vi "3090仪器参数上传.vi"(11 "错误输入（无错误）":errorcluster) -> (15 "error out":errorcluster)   [LabVIEW 2016, in "数据传输系统.lvlib"]
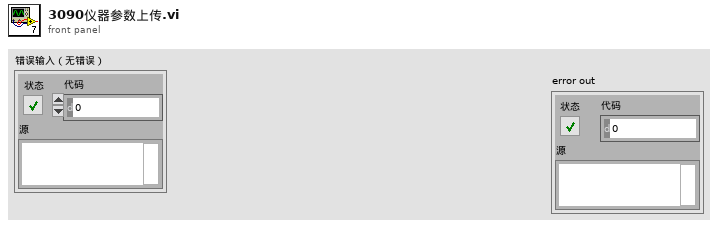
[diagram p1: front panel]
types:
  T1 = cluster{"氨氮仪器参数索引起始时间":string, "总磷仪器参数索引起始时间":string, "总氮仪器参数索引起始时间":string, "CODMn仪器参数索引起始时间":string, "CODCr仪器参数索引起始时间":string, "DO仪器参数索引起始时间":string, "PH仪器参数索引起始时间":string, "比电导率仪器参数索引起始时间":string, "水温仪器参数索引起始时间":string, "浊度仪器参数索引起始时间":string, "叶绿素a仪器参数索引起始时间":string, "藻密度仪器参数索引起始时间":string, "ORP仪器参数索引起始时间":string}
  T2 = cluster{"[0]":string, "[1]":string, "[2]":string, "[3]":string, "[4]":string, "[5]":string, "[6]":string, "[7]":string, "[8]":string, "[9]":string, "[10]":string, "[11]":string, "[12]":string}
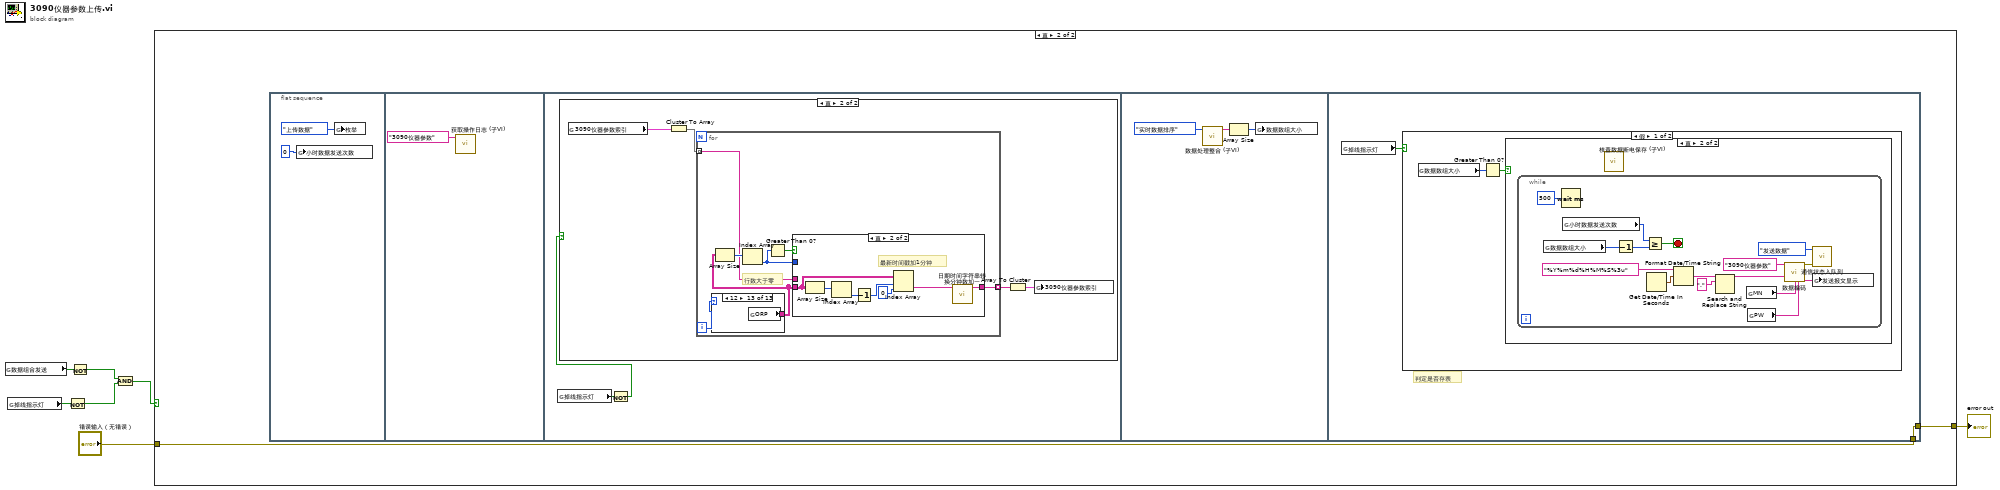
[diagram p0: block diagram]
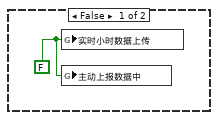
[diagram p2: hidden frame]
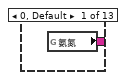
[diagram p4: hidden frame]
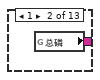
[diagram p5: hidden frame]
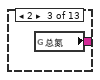
[diagram p6: hidden frame]
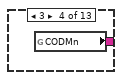
[diagram p7: hidden frame]
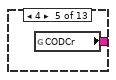
[diagram p8: hidden frame]
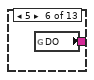
[diagram p9: hidden frame]
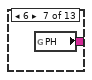
[diagram p10: hidden frame]
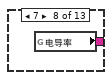
[diagram p11: hidden frame]
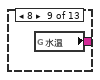
[diagram p12: hidden frame]
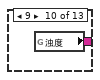
[diagram p13: hidden frame]
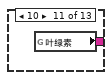
[diagram p14: hidden frame]
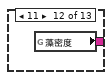
[diagram p15: hidden frame]
diagram:
  n1 = global read "断电保存全局.vi" "数据组合发送"() -> (w4:bool)
  n2 = global read "全局 数据发送重叠.vi" "掉线指示灯"() -> (w7:bool)
  n3 = Not(x=w7) -> (.not. x?=w2:bool)
  n4 = Not(x=w4) -> (.not. x?=w3:bool)
  n5 = And(x=w3, y=w2) -> (x .and. y?=w1:bool)
  n6 = case shown="真" w1 {
    tunnel: [_ w10] -> w6
    tunnel: "错误输入（无错误）" -> [_ w9]
    frame False {
      w8 = FALSE ("小时数据上传")
      n7 = global write "全局1.vi" "实时小时数据上传"(w8) -> ()
      n8 = global write "全局 数据发送重叠.vi" "主动上报数据中"(w8) -> ()
    }
    frame True {
      n9 = flat-sequence {
        tunnel: [w51] -> w10
        tunnel: w9 -> [w51]
        frame #0 {
          n10 = global write "全局 小时数据发送次数.vi" "小时数据发送次数"(0 ("小时数据发送次数")) -> ()
          n11 = global write "全局1.vi" "枚举"(enum16{"返回请求应答", "上传数据", "返回执行结果"}."上传数据" ("枚举")) -> ()
        }
        frame #1 {
          n12 = call "获取操作日志 (子VI).vi"("table输入"="3090仪器参数") -> ()  [unwired: 11 in]
        }
        frame #2 {
          n13 = global read "全局 数据发送重叠.vi" "掉线指示灯"() -> (w15:bool)
          n14 = Not(x=w15) -> (.not. x?=w14:bool)
          n15 = case shown="真" w14 {
            frame False {
            }
            frame True {
              n16 = global read "全局 时间2.vi" "3090仪器参数索引"() -> (w19:T1)
              n17 = Cluster To Array(cluster=w19) -> (array=w18:string[])
              n18 = for {
                tunnel: [w23] -> w16 mode=indexing
                tunnel: w18 -> [w22] mode=indexing
                i -> [w21]
                # "行数大于零"
                n19 = case shown="12" w21 {
                  tunnel: [w27 w28 w29 w30 w31 w32 w33 w34 w35 w36 w37 w38 w39] -> w20
                  frame 0, Default {
                    n20 = global read "全局 所有参数.vi" "氨氮"() -> (w27:string[][])
                  }
                  frame 1 {
                    n21 = global read "全局 所有参数.vi" "总磷"() -> (w28:string[][])
                  }
                  frame 2 {
                    n22 = global read "全局 所有参数.vi" "总氮"() -> (w29:string[][])
                  }
                  frame 3 {
                    n23 = global read "全局 所有参数.vi" "CODMn"() -> (w30:string[][])
                  }
                  frame 4 {
                    n24 = global read "全局 所有参数.vi" "CODCr"() -> (w31:string[][])
                  }
                  frame 5 {
                    n25 = global read "全局 所有参数.vi" "DO"() -> (w32:string[][])
                  }
                  frame 6 {
                    n26 = global read "全局 所有参数.vi" "PH"() -> (w33:string[][])
                  }
                  frame 7 {
                    n27 = global read "全局 所有参数.vi" "电导率"() -> (w34:string[][])
                  }
                  frame 8 {
                    n28 = global read "全局 所有参数.vi" "水温"() -> (w35:string[][])
                  }
                  frame 9 {
                    n29 = global read "全局 所有参数.vi" "浊度"() -> (w36:string[][])
                  }
                  frame 10 {
                    n30 = global read "全局 所有参数.vi" "叶绿素"() -> (w37:string[][])
                  }
                  frame 11 {
                    n31 = global read "全局 所有参数.vi" "藻密度"() -> (w38:string[][])
                  }
                  frame 12 {
                    n32 = global read "全局 所有参数.vi" "ORP"() -> (w39:string[][])
                  }
                }
                n33 = Array Size(array=w20) -> (size(s)=w25:i32[])
                n34 = Index Array(array=w25) -> (element=w24:i32)  [unwired: 1 in]
                n35 = Greater Than 0?(x=w24) -> (x > 0?=w26:bool)
                n36 = case shown="真" w26 {
                  tunnel: w24 -> [_ _]
                  tunnel: w20 -> [_ w44]
                  tunnel: [w40 w41] -> w23
                  tunnel: w22 -> [w40 _]
                  frame False {
                  }
                  frame True {
                    # "最新时间戳加1分钟"
                    n37 = Array Size(array=w44) -> (size(s)=w46:i32[])
                    n38 = Index Array(array=w46) -> (element=w45:i32)  [unwired: 1 in]
                    n39 = Decrement(x=w45) -> (x-1=w43:i32)
                    n40 = Index Array(array=w44, index (row)=w43, index (col)=0 ("禁用的索引 (列)")) -> (element=w47:string)
                    n41 = call "日期时间字符串转换分钟数加一.vi"("data[0]"=w47) -> ("日期/时间字符串"=w41:string)  [unwired: 10 in]
                  }
                }
              }
              n42 = Array To Cluster(array=w16) -> (cluster=w17:T2)
              n43 = global write "全局 时间2.vi" "3090仪器参数索引"(w17) -> ()
            }
          }
        }
        frame #3 {
          n44 = call "数据处理整合 (子VI).vi"("枚举"=enum16{"实时数据排序", "小时数据排序"}."实时数据排序") -> ("已排序的数组"=w50:string[])  [unwired: 10 in]
          n45 = Array Size(array=w50) -> (size(s)=w49:i32)
          n46 = global write "全局 数据数组大小.vi" "数据数组大小"(w49) -> ()
        }
        frame #4 {
          # "判定是否存表"
          n47 = global read "全局 数据发送重叠.vi" "掉线指示灯"() -> (w52:bool)
          n48 = case shown="假" w52 {
            frame False {
              n49 = global read "全局 数据数组大小.vi" "数据数组大小"() -> (w53:i32)
              n50 = Greater Than 0?(x=w53) -> (x > 0?=w54:bool)
              n51 = case shown="真" w54 {
                frame False {
                }
                frame True {
                  n52 = while {
                    stop <- w55 stop-if-true
                    n53 = global read "全局 数据数组大小.vi" "数据数组大小"() -> (w57:i32)
                    n54 = Wait (ms)(milliseconds to wait=u32 500 ("等待时间（毫秒）")) -> ()  [unwired: 1 out]
                    n55 = global read "全局 小时数据发送次数.vi" "小时数据发送次数"() -> (w58:i32)
                    n56 = Decrement(x=w57) -> (x-1=w56:i32)
                    n57 = Greater Or Equal?(x=w58, y=w56) -> (x >= y?=w55:bool)
                    n58 = Get Date/Time In Seconds() -> (seconds since 1Jan1904=w68:timestamp)
                    n59 = Format Date/Time String(time format string (%c)="%Y%m%d%H%M%S%3u" ("时间格式字符串(%c)"), seconds (now)=w68) -> (date/time string=w67:string)  [unwired: 1 in]
                    n60 = Search and Replace String(input string=w67, search string="." ("搜索字符串")) -> (result string=w65:string)  [unwired: 6 in, 3 out]
                    n61 = global read "断电保存全局.vi" "MN"() -> (w62:string)
                    n62 = global read "断电保存全局.vi" "PW"() -> (w61:string)
                    n63 = call "数据编码.vi"("table输入"="3090仪器参数" ("新元素/子数组"), "QN"=w65, "MN"=w62, "PW"=w61) -> ("错误常量"=w60:errorcluster, "通讯包字符串"=w64:string)  [unwired: 10 in]
                    n64 = call "通信状态入队列.vi"("错误输入（无错误）"=w60, "枚举"=enum16{"打开连接", "发送数据", "读取数据", "数据处理", "关闭连接"}."发送数据") -> ()  [unwired: 9 in, 1 out]
                    n65 = global write "全局1.vi" "发送报文显示"(w64) -> ()
                  }
                  n66 = call "核查数据断电保存 (子VI).vi"() -> ()  [unwired: 12 in]
                }
              }
            }
            frame True {
            }
          }
        }
      }
    }
  }
  "error out" <- w6
